vi "main.vi"() -> ()   [LabVIEW 2009]
uses:
  typedefs/ScanAxisCfg.ctl
  typedefs/AxisSelect_Enum.ctl
  typedefs/SweepMode_Ring.ctl
  typedefs/ScanType.ctl
  typedefs/DwellTime.ctl
  typedefs/PathCluster.ctl
  typedefs/main_States.ctl
  globals/VISAResourceName.vi
  typedefs/AxisSpaceCfg.ctl
  typedefs/AxisCfg.ctl
  globals/AxisSpace.vi
  typedefs/Ultra3000/Index_Numeric.ctl
  typedefs/Ultra3000/HostControlModeRing.ctl
  typedefs/Ultra3000/IndexType.ctl
  typedefs/Ultra3000/IndexSettings_Cluster.ctl
panel:
  in  "Move to index stop":bool
  in  "Move to index start":bool
  in  "Move to scan stop":bool
  in  "Move to scan start":bool
  in  "Scan Axis":T1
  in  "Same as Scan Axis":bool
  in  "Index Axis":T1={"Axis "=enum."Y", "Velocity"=0.0, "Accel./Decel."=0.0, "Deadband"=0.0, "Start Position"=0.0, "Total Length"=0.0, "Stop Position"=0.0, "Pixel Increment"=0.0}
  in  "File Paths":T3
  in  "Scan Options":T7
  in  "open":bool
  in  "Tools":T8(ring)
  in  "Exit":bool
  in  "Start Scan":bool
  # "Scan Configuration"
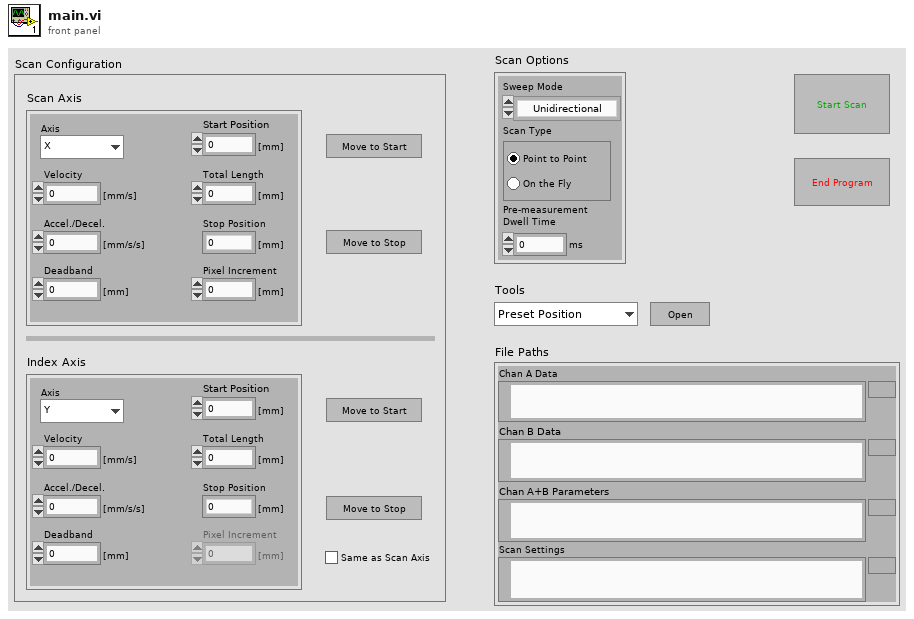
[diagram p1: front panel]
types:
  T1 = typedef "ScanAxisCfg.ctl" = cluster{"Axis ":T2, "Velocity":dbl, "Accel./Decel.":dbl, "Deadband":dbl, "Start Position":dbl, "Total Length":dbl, "Stop Position":dbl, "Pixel Increment":dbl}
  T2 = typedef "AxisSelect_Enum.ctl" = enum16{"X", "Y", "Z", "Axis Space"}
  T3 = typedef "PathCluster.ctl" = cluster{"Chan A Data":path, "Chan B Data":path, "Chan A+B Parameters":path, "Scan Settings":path}
  T4 = typedef "SweepMode_Ring.ctl" = enum16{"Unidirectional", "Bidirectional"}
  T5 = typedef "ScanType.ctl" = enum32{"Point to Point", "On the Fly"}
  T6 = typedef "DwellTime.ctl" = u16
  T7 = cluster{"Sweep Mode":T4, "Scan Type":T5, "Pre-measurement\nDwell Time":T6}
  T8 = enum16{"Preset Position", "Axis Settings", "Test Axes"}
  T9 = typedef "main_States.ctl" = enum16{"Handle FP Events", "Same as Scan Axis", "Exit", "Axis Start", "Open Tools", "Update Stop Position", "Start Scan", "Axis Stop", "Initialize Scanner", "Abort", "Connect Serial Port", "Initialize", "Export", "Import"}
  T10 = enum16{"open", "replace", "create", "open or create", "replace or create", "replace or create with confirmation"}
  T11 = typedef "Index_Numeric.ctl" = u8
  T12 = enum8{"Enabled", "Disabled", "Disabled and Grayed Out"}
  T13 = typedef "IndexSettings_Cluster.ctl" = cluster{"Type":T14, "Dwell":T6, "Velocity":dbl, "Accel/Decel":dbl}
  T14 = typedef "IndexType.ctl" = i32
  T15 = typedef "AxisSpaceCfg.ctl" = T16[]
  T16 = typedef "AxisCfg.ctl" = cluster{"Addr":u8, "Conv Factor":dbl, "Forward Limit":dbl, "Reverse Limit":dbl, "Enable Limits":bool}
  T17 = typedef "HostControlModeRing.ctl" = u16
  T18 = typedef "ReplaySettings.ctl" = cluster{"Sampling Rate":dbl, "Samples in replay":u32, "Replay Start Time":dbl, "Replay Stop Time":dbl}
  T19 = typedef "Acquire Event type.ctl" = cluster{"Acquire Mode":T20, "Acquisition mode":T21, "Acquirer":T22, "Transfer Chans":enum16{"Chan A", "Chan B", "Chan A+B"}, "A max scale":dbl, "A min scale":dbl, "B max scale":dbl, "B min scale":dbl, "A Probe":T23, "B Probe":T23, "A Coupling":T24, "B Coupling":T24, "A Bandwidth":T25, "B Bandwidth":T25, "Trigger Source":T26, "Trigger Amplitude":dbl, "A Trigger Amplitude":dbl, "B Trigger Amplitude":dbl, "Trigger Filter":T27, "Trig Slope":bool, "Trigger Holdoff":dbl, "Dig Pattern Rqd":bool, "Dig Pattern":u32, "Ext Trig Threshold":dbl, "Dig Input Threshold":dbl, "Start Time":dbl, "Stop Time":dbl, "Pre Trig Time":dbl, "Port":enum16{"Port 1", "Port 2", "Port 3", "Port 4", "Port 5", "Port 6"}, "Num divisions":i16, "Num seq frames":i16, "Num Buffers":i32, "Sig Gen Freq":dbl, "Sig Gen Amp":dbl, "Sig Gen Offset":dbl, "Sig Gen Waveform":T28, "Sig Gen Sweep":enum16{"Linear", "Log"}, "Sig Gen Func":enum16{"Standard", "Auto advance", "Freq mod In8", "Phase mod In8"}, "Sig Gen Freq 2":dbl, "Sig Gen Phase":dbl, "Trig 2 Function":T29, "Min Trigger Period":dbl, "Max trigger Period":dbl, "Trigger count":u32, "Trig 2 Slope":bool, "Trig 2 Source Chan":T30, "Trig 2 Level":dbl, "Dig Pattern 2 Rqd":bool, "Dig Pattern 2":u32, "Trigger 2 Source":enum16{"Trigger 1 inverted", "Trig 2 Defn"}, "Waveform Averages":i32, "Value changed":i32, "Freq Span":dbl, "Freq Res":dbl, "Duration":dbl, "Resolution":dbl, "Link Port":T31, "Ext Sample Clock":bool, "F Spare 2":bool, "F Spare 3":bool, "F Spare 4":bool, "Sampler Resolution":T32, "Intf Source":T33, "Update Rate":enum16{"20 Frame/sec", "10 Frame/sec", "5 Frame/sec"}, "Transfer Size":T34, "Sig Gen Freq Step":dbl, "TCP Adr":u32, "TCP port":u32, "CAU Ser Num Hi":u32, "CAU Ser Num Lo":u32, "Function Number":dbl, "Function Parameter":dbl, "Function Result":dbl, "Link Start":u32, "Link Timebase":u32, "Link Timer":u32, "Link Setup":u32, "Spare 1":dbl, "Spare 2":dbl, "Spare 3":dbl, "Spare 4":dbl}
  T20 = typedef "Acquire capture type.ctl" = enum16{"single", "automatic", "triggered", "stop", "single stop", "replay"}
  T21 = typedef "Acquire capture method.ctl" = enum16{"Sampled", "Peak Captured", "Filtered", "Repetitive", "Waveform avg"}
  T22 = typedef "Acquirer type.ctl" = enum16{"Internal Sig Gen", "APC 901", "APC 901A", "Sound Card", "Cleverscope"}
  T23 = typedef "Input Range.ctl" = enum16{"x1", "x10", "x100", "x1K", "x20", "x50", "x200"}
  T24 = typedef "Input Coupling.ctl" = enum16{"AC", "DC"}
  T25 = typedef "Input Bandwidth.ctl" = u16
  T26 = typedef "USB channel.ctl" = enum32{"Chan A", "Chan B", "Ext Trigger", "Dig Trig", "Link Input", "chan_5", "chan_6", "chan_7", "chan_8", "chan_9", "chan_10", "chan_11", "chan_12", "chan_13", "chan_14", "chan_15"}
  T27 = typedef "Trigger Filter.ctl" = enum16{"None", "Low Pass", "Hi Pass", "Noise"}
  T28 = typedef "Cscope waveform type.ctl" = enum16{"sine", "triangle", "square", "DC", "OFF"}
  T29 = typedef "Trigger Period.ctl" = enum16{"None", "Trig 1~2 < min", "min<T1~2 < max", "Trig 1~2 > max", "Count Trig 1", "Count Trig 2"}
  T30 = typedef "Trigger channel.ctl" = enum32{"Chan A", "Chan B", "Ext Trigger", "Dig Trig", "Link Input"}
  T31 = typedef "Link port types.ctl" = enum8{"Debug", "Link Out", "Disabled", "Slave", "Master", "Uart", "SPI", "I2C", "Digital", "Sig Gen"}
  T32 = typedef "Acquirer resolution.ctl" = enum16{"10 bit", "12 Bit", "14 bit"}
  T33 = typedef "Intf source.ctl" = enum16{"USB", "Ethernet - Find by IP address", "Ethernet - Find first IP address", "Ethernet - Find by serial number"}
  T34 = typedef "Acquire transfer size.ctl" = enum16{"Normal", "100% Buffer", "50% Buffer", "10% Buffer", "5% Buffer", "2% Buffer", "Sequence"}
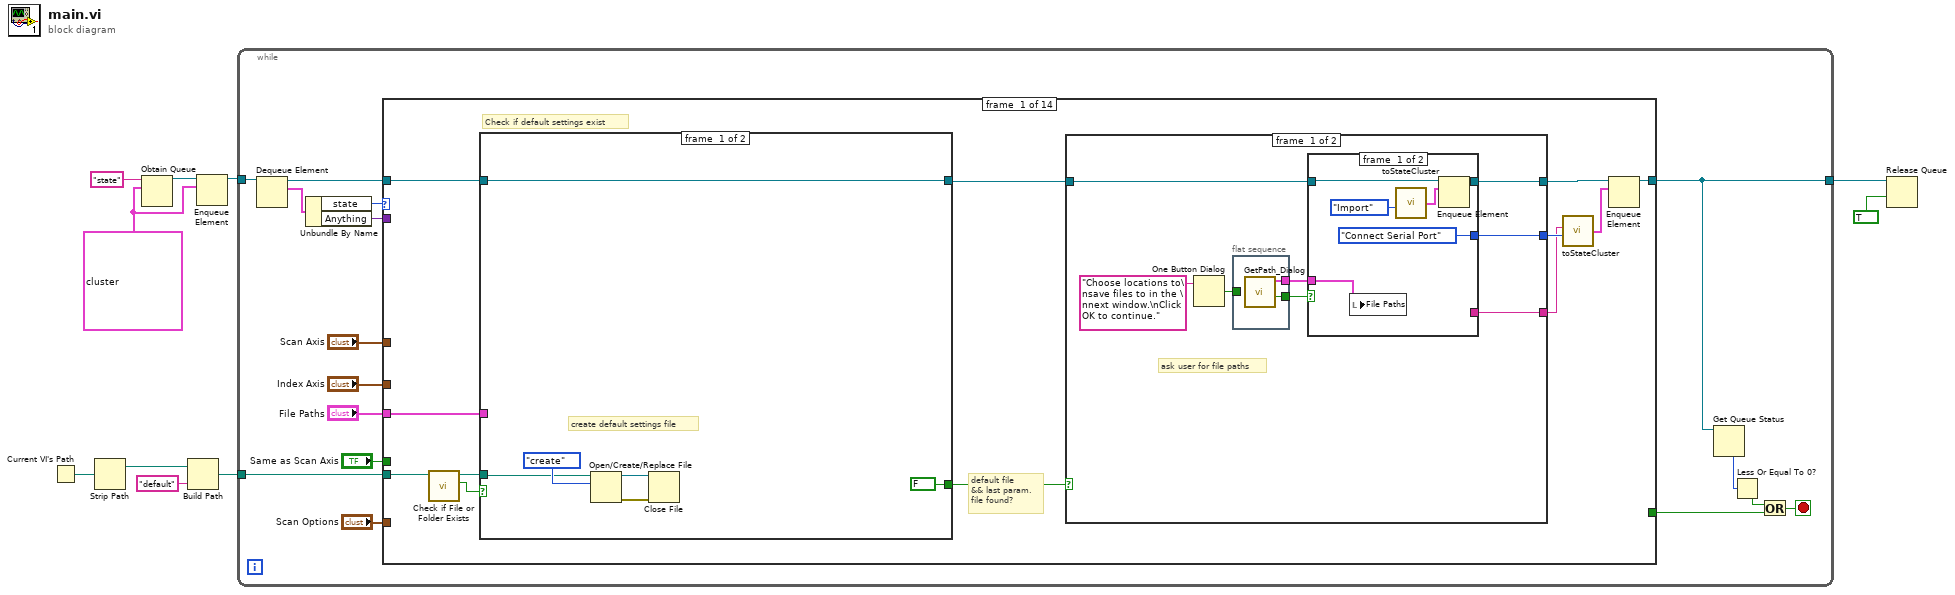
[diagram p0: block diagram]
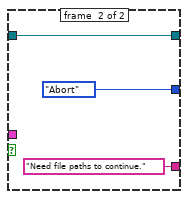
[diagram p2: hidden frame]
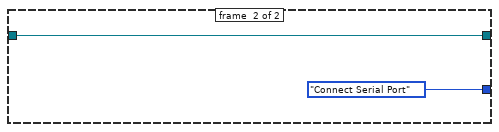
[diagram p3: hidden frame]
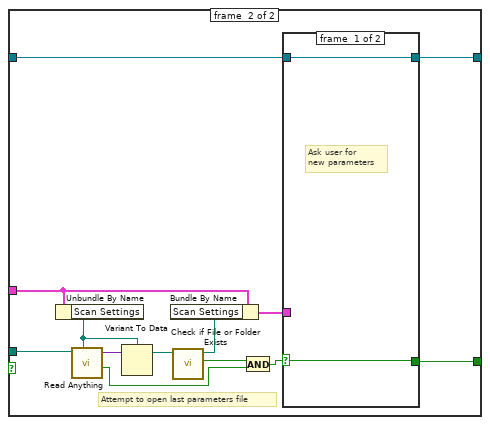
[diagram p4: hidden frame]
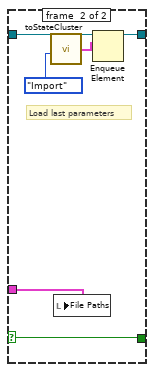
[diagram p5: hidden frame]
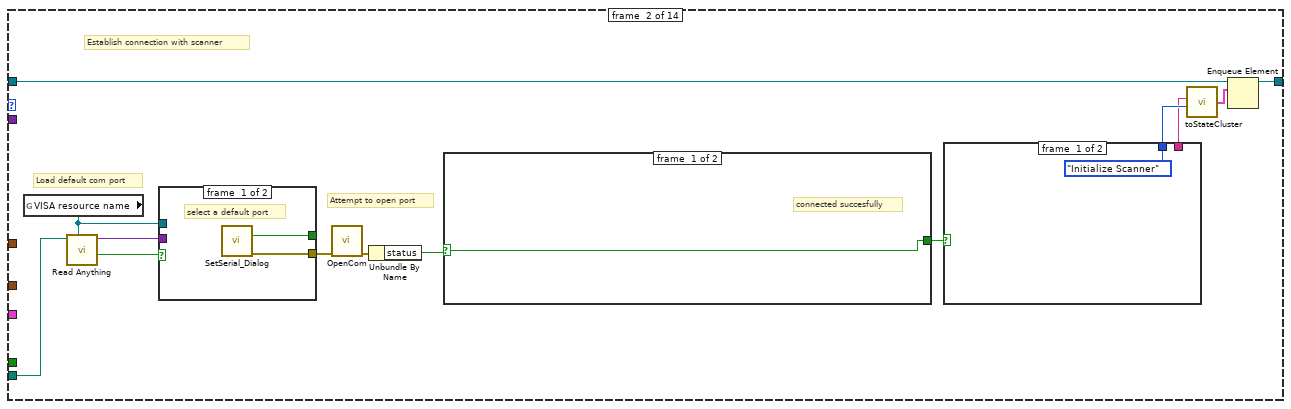
[diagram p6: hidden frame]
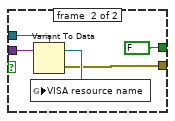
[diagram p7: hidden frame]
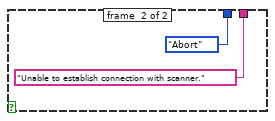
[diagram p8: hidden frame]
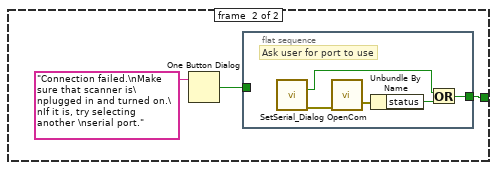
[diagram p9: hidden frame]
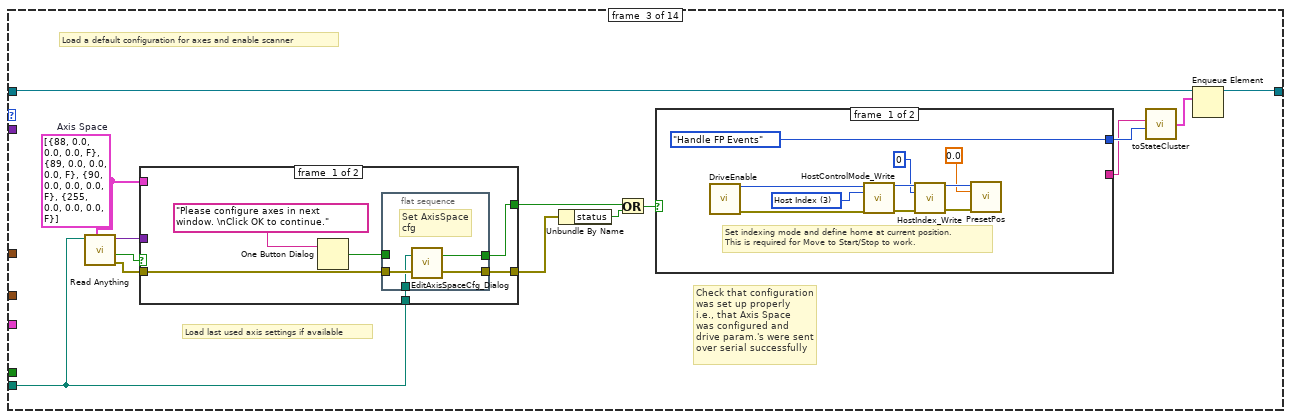
[diagram p10: hidden frame]
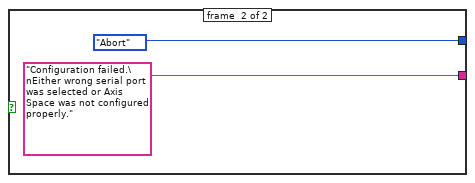
[diagram p11: hidden frame]
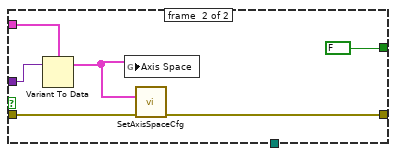
[diagram p12: hidden frame]
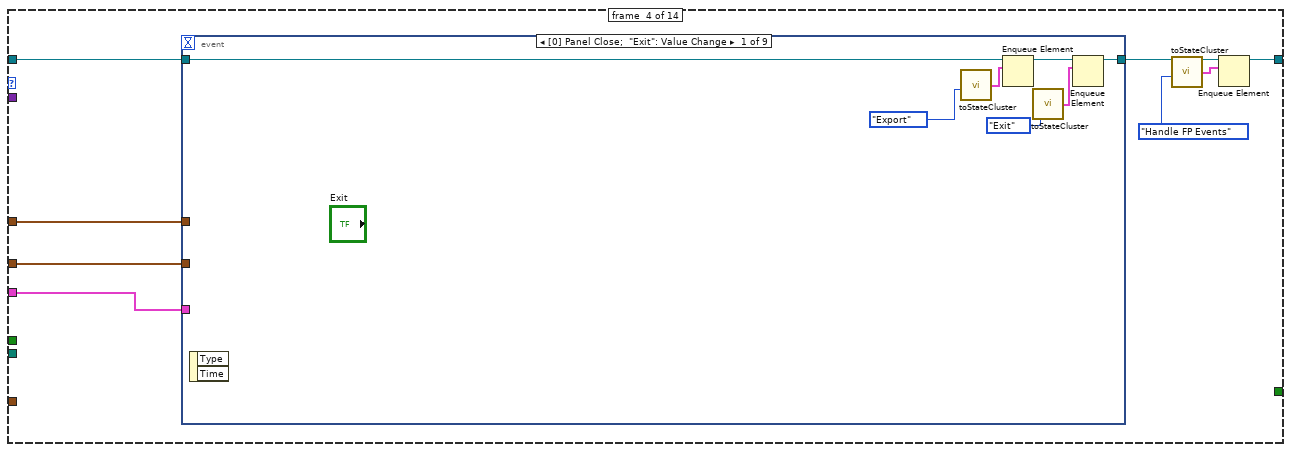
[diagram p13: hidden frame]
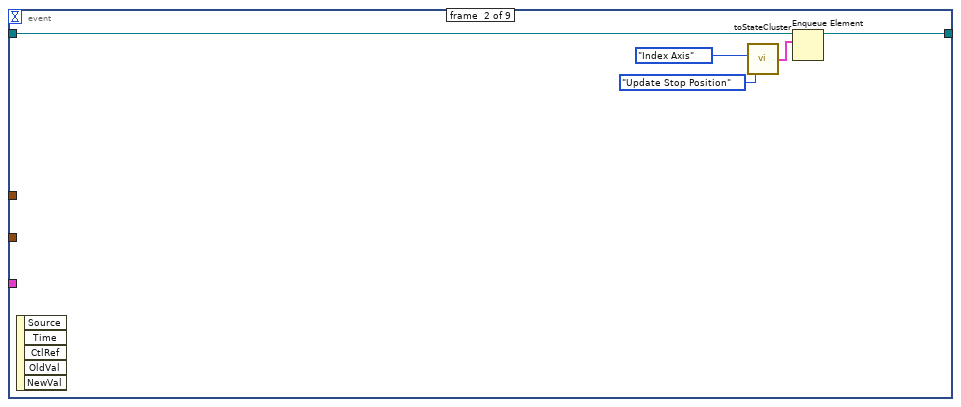
[diagram p14: hidden frame]
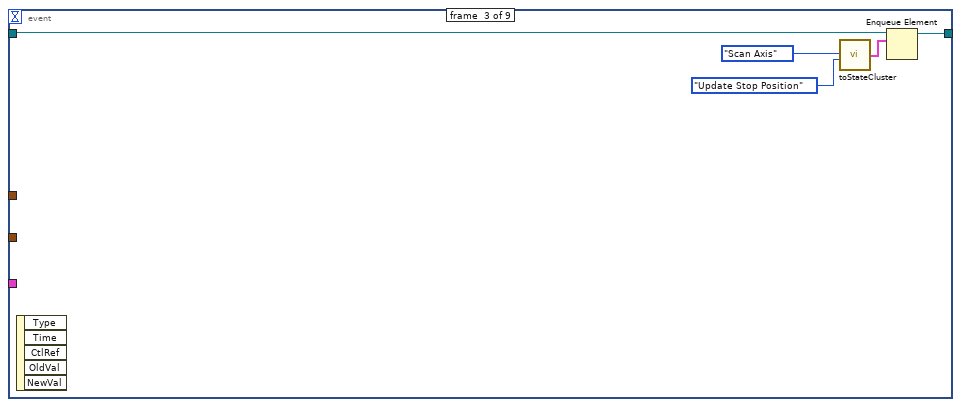
[diagram p15: hidden frame]
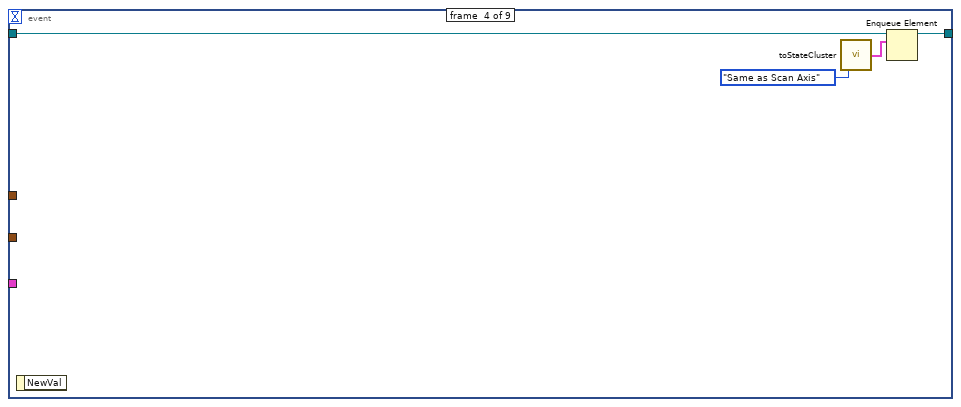
[diagram p16: hidden frame]
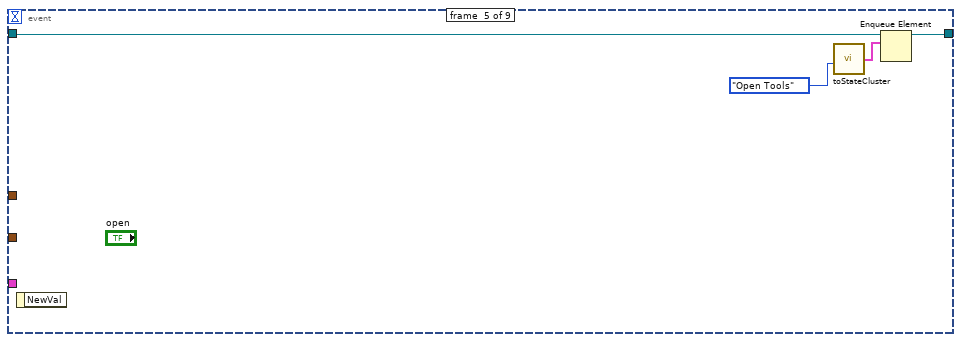
[diagram p17: hidden frame]
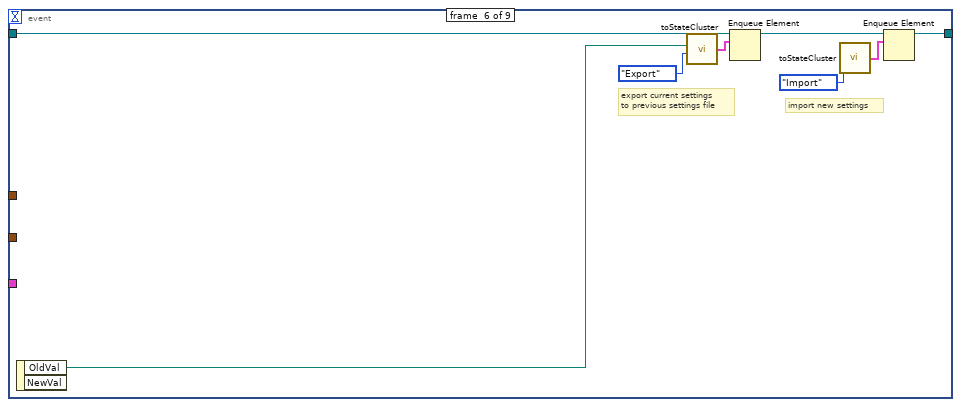
[diagram p18: hidden frame]
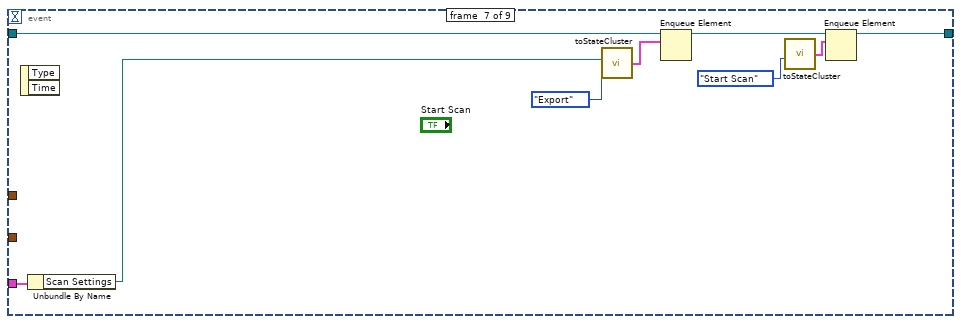
[diagram p19: hidden frame]
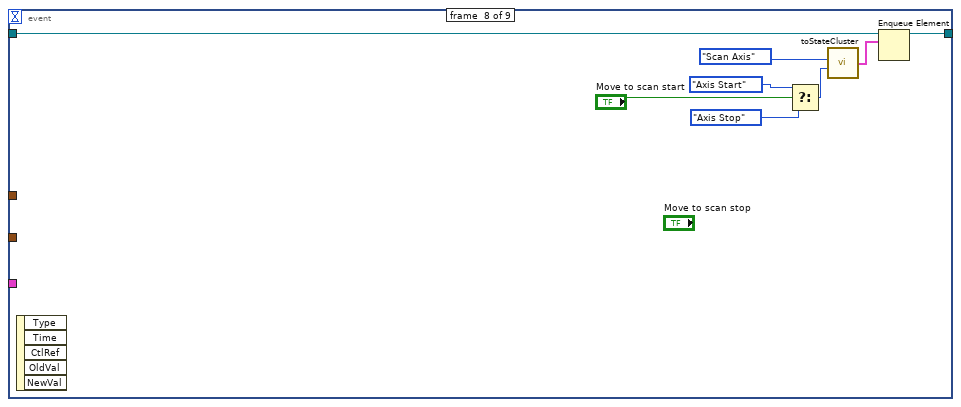
[diagram p20: hidden frame]
diagram:
  w1 = cluster{"Anything":variant, "state":T9} {"Anything"=variant, "state"=enum."Initialize"}
  n1 = Current VI's Path() -> (path=w3:path)
  n2 = Strip Path(path=w3) -> (stripped path=w2:path)  [unwired: 1 out]
  n3 = Obtain Queue(name (unnamed)="state", element data type=w1) -> (queue out=w7:refnum<queue>)  [unwired: 3 in, 2 out]
  n4 = Build Path(base path=w2, name or relative path="default") -> (appended path=w4:path)
  n5 = Enqueue Element(queue=w7, element=w1) -> (queue out=w6:refnum<queue>)  [unwired: 2 in, 2 out]
  n6 = while {
    tunnel: w6 -> [w22]
    tunnel: [w16] -> w9
    tunnel: w4 -> [w15]
    stop <- w20 stop-if-true
    n7 = Dequeue Element(queue=w22) -> (queue out=w21:refnum<queue>, element=w13:cluster{"Anything":variant, "state":T9})  [unwired: 2 in, 2 out]
    n8 = Unbundle By Name(w13) -> ("state"=w12:T9, "Anything"=w11:variant)
    n9 = case shown="\"Connect Serial Port\"" w12 {
      tunnel: "Scan Axis" -> [_ _ _ w168 w231 w244 w259 w275 _ w295 _ _ w348 w370]
      tunnel: [_ _ _ _ _ _ _ _ _ _ TRUE ("Exit") TRUE ("Exit") _ _] -> w19
      tunnel: "Index Axis" -> [_ _ _ w167 w233 _ w260 w276 _ w293 _ _ w347 w369]
      tunnel: "File Paths" -> [w36 _ _ w166 _ _ _ _ _ w294 _ w326 w340 w361]
      tunnel: "Scan Options" -> [_ _ _ _ _ _ _ _ _ w291 _ _ w346 w371]
      tunnel: w21 -> [w34 w97 w128 w165 w230 w243 w257 w273 w287 w290 w321 w329 w351 w366]
      tunnel: [w32 w98 w127 w164 w230 w243 w257 w273 w287 w290 w321 w329 w351 w367] -> w16
      tunnel: w15 -> [w38 w92 w122 _ _ _ _ _ w286 _ _ w324 _ _]
      tunnel: "Same as Scan Axis" -> [_ _ _ _ _ w242 _ _ _ _ _ _ w345 w365]
      tunnel: w11 -> [_ _ _ _ w229 _ w255 w271 _ _ w320 _ w333 w357]
      frame #0 {
        # "default file\n&& last param.\nfile found?"
        # "Check if default settings exist"
        n10 = call <vilib>:"Check if File or Folder Exists.vi"("path"=w38) -> ("file or folder exists?"=w37:bool, "dup path"=w35:path)  [unwired: 8 in, 1 out]
        n11 = case shown="True" w37 {
          tunnel: w36 -> [_ w77]
          tunnel: w35 -> [w62 w71]
          tunnel: w34 -> [w61 w72]
          tunnel: [w61 w73] -> w31
          tunnel: [FALSE w70] -> w30
          frame #0 {
            # "create default settings file"
            n12 = Open/Create/Replace File(file path (use dialog)=w62, operation (0:open)=T10."create") -> (refnum out=w64:refnum<file>, error out=w63:errorcluster)  [unwired: 4 in, 1 out]
            n13 = Close File(refnum=w64, error in=w63) -> ()  [unwired: 2 out]
          }
          frame #1 {
            # "Attempt to open last parameters file"
            n14 = Unbundle By Name(w77) -> ("Scan Settings"=w76:path)
            n15 = call "Read Anything.vi"("Type of Anything"=w76, "Path (dialog)"=w71) -> ("Found?"=w66:bool, "Anything"=w78:variant)  [unwired: 7 in, 1 out]
            n16 = Variant To Data(Variant=w78, type=w76) -> (data=w74:path)  [unwired: 1 in, 1 out]
            n17 = call <vilib>:"Check if File or Folder Exists.vi"("path"=w74) -> ("file or folder exists?"=w67:bool, "dup path"=w69:path)  [unwired: 8 in, 1 out]
            n18 = Bundle By Name(cluster=w77, "Scan Settings"=w69) -> (w75:T3)
            n19 = And(x=w67, y=w66) -> (x .and. y?=w68:bool)
            n20 = case shown="True" w68 {
              selector: w68 -> [w79 w83]
              tunnel: w75 -> [_ w86]
              tunnel: [w80 w85] -> w73
              tunnel: w72 -> [w80 w84]
              tunnel: [w79 w83] -> w70
              frame #0 {
                # "Ask user for \nnew parameters"
              }
              frame #1 {
                # "Load last parameters"
                n21 = call "toStateCluster.vi"("state"=main_States."Import" ("element")) -> ("output cluster"=w82:cluster{"Anything":variant, "state":T9})  [unwired: 5 in]
                n22 = local write "File Paths"(w86) -> ()
                n23 = Enqueue Element(queue=w84, element=w82) -> (queue out=w85:refnum<queue>)  [unwired: 2 in, 2 out]
              }
            }
          }
        }
        n24 = case shown="True" w30 {
          tunnel: [w42 _] -> w27
          tunnel: [w40 w59] -> w33
          tunnel: w31 -> [w41 w59]
          tunnel: [w39 main_States."Connect Serial Port"] -> w29
          frame #0 {
            # "ask user for file paths"
            n25 = One Button Dialog(message="Choose locations to\nsave files to in the \nnext window.\nClick OK to continue.") -> (true=w43:bool)  [unwired: 1 in]
            n26 = flat-sequence {
              tunnel: [w48] -> w46
              tunnel: [w47] -> w45
              tunnel: w43 -> [_]
              frame #0 {
                n27 = call "GetPath_Dialog.vi"() -> ("Cancelled?"=w48:bool, "File Paths Out"=w47:T3)  [unwired: 10 in]
              }
            }
            n28 = case shown="False" w46 {
              tunnel: [_ "Need file paths to continue." ("message")] -> w42
              tunnel: w45 -> [w54 _]
              tunnel: [w52 w56] -> w40
              tunnel: w41 -> [w51 w56]
              tunnel: [main_States."Connect Serial Port" main_States."Abort"] -> w39
              frame #0 {
                n29 = local write "File Paths"(w54) -> ()
                n30 = call "toStateCluster.vi"("state"=main_States."Import" ("element")) -> ("output cluster"=w50:cluster{"Anything":variant, "state":T9})  [unwired: 5 in]
                n31 = Enqueue Element(queue=w51, element=w50) -> (queue out=w52:refnum<queue>)  [unwired: 2 in, 2 out]
              }
              frame #1 {
              }
            }
          }
          frame #1 {
          }
        }
        n32 = call "toStateCluster.vi"("state"=w29, "Anything"=w27) -> ("output cluster"=w28:cluster{"Anything":variant, "state":T9})  [unwired: 4 in]
        n33 = Enqueue Element(queue=w33, element=w28) -> (queue out=w32:refnum<queue>)  [unwired: 2 in, 2 out]
      }
      frame #1 {
        # "Establish connection with scanner"
        # "Load default com port"
        # "Attempt to open port"
        n34 = global read "VISAResourceName.vi" "VISA resource name"() -> (w93:refnum<visa-resource-name>)
        n35 = call "Read Anything.vi"("Type of Anything"=w93, "Path (dialog)"=w92) -> ("Found?"=w91:bool, "Anything"=w94:variant)  [unwired: 7 in, 1 out]
        n36 = case shown="True" w91 {
          tunnel: w94 -> [_ w106]
          tunnel: w93 -> [_ w104]
          tunnel: [w101 FALSE ("Cancelled?")] -> _
          tunnel: [w100 w102] -> w90
          frame #0 {
            # "select a default port"
            n37 = call "SetSerial_Dialog.vi"() -> ("Cancelled?"=w101:bool, "error out"=w100:errorcluster)  [unwired: 14 in]
          }
          frame #1 {
            n38 = Variant To Data(Variant=w106, type=w104) -> (error out=w102:errorcluster, data=w105:refnum<visa-resource-name>)  [unwired: 1 in]
            n39 = global write "VISAResourceName.vi" "VISA resource name"(w105) -> ()
          }
        }
        n40 = call "OpenCom.vi"("error in (no error)"=w90) -> ("error out"=w96:errorcluster)  [unwired: 14 in]
        n41 = Unbundle By Name(w96) -> ("status"=w95:bool)
        n42 = case shown="True" w95 {
          selector: w95 -> [w110 _]
          tunnel: [w110 w113] -> w99
          frame #0 {
            # "connected succesfully"
          }
          frame #1 {
            n43 = One Button Dialog(message="Connection failed.\nMake sure that scanner is\nplugged in and turned on.\nIf it is, try selecting another \nserial port.") -> (true=w112:bool)  [unwired: 1 in]
            n44 = flat-sequence {
              tunnel: [w118] -> w113
              tunnel: w112 -> [_]
              frame #0 {
                # "Ask user for port to use"
                n45 = call "SetSerial_Dialog.vi"() -> ("Cancelled?"=w117:bool, "error out"=w116:errorcluster)  [unwired: 14 in]
                n46 = call "OpenCom.vi"("error in (no error)"=w116) -> ("error out"=w115:errorcluster)  [unwired: 14 in]
                n47 = Unbundle By Name(w115) -> ("status"=w114:bool)
                n48 = Or(x=w117, y=w114) -> (x .or. y?=w118:bool)
              }
            }
          }
        }
        n49 = case shown="False" w99 {
          tunnel: [main_States."Initialize Scanner" main_States."Abort"] -> w89
          tunnel: [_ "Unable to establish connection with scanner." ("message")] -> w87
          frame #0 {
          }
          frame #1 {
          }
        }
        n50 = call "toStateCluster.vi"("state"=w89, "Anything"=w87) -> ("output cluster"=w88:cluster{"Anything":variant, "state":T9})  [unwired: 4 in]
        n51 = Enqueue Element(queue=w97, element=w88) -> (queue out=w98:refnum<queue>)  [unwired: 2 in, 2 out]
      }
      frame #2 {
        w125 = T15 [{"Addr"=88, "Conv Factor"=0.0, "Forward Limit"=0.0, "Reverse Limit"=0.0, "Enable Limits"=FALSE}, {"Addr"=89, "Conv Factor"=0.0, "Forward Limit"=0.0, "Reverse Limit"=0.0, "Enable Limits"=FALSE}, {"Addr"=90, "Conv Factor"=0.0, "Forward Limit"=0.0, "Reverse Limit"=0.0, "Enable Limits"=FALSE}, {"Addr"=255, "Conv Factor"=0.0, "Forward Limit"=0.0, "Reverse Limit"=0.0, "Enable Limits"=FALSE}]  # Axis Space
        # "Load a default configuration for axes and enable scanner"
        # "Check that configuration\nwas set up properly\ni.e., that Axis Space\nwas configured and \ndrive param.'s were sent\nover serial successfully"
        # "Load last used axis settings if available"
        n52 = call "Read Anything.vi"("Type of Anything"=w125, "Path (dialog)"=w122) -> ("Error Out"=w124:errorcluster, "Found?"=w123:bool, "Anything"=w126:variant)  [unwired: 7 in]
        n53 = case shown="True" w123 {
          tunnel: [w150 FALSE ("Cancelled?")] -> w129
          tunnel: [w149 w159] -> w132
          tunnel: w124 -> [w148 w158]
          tunnel: w126 -> [_ w157]
          tunnel: w125 -> [_ w156]
          tunnel: w122 -> [w147 _]
          frame #0 {
            n54 = One Button Dialog(message="Please configure axes in next window. \nClick OK to continue.") -> (true=w145:bool)  [unwired: 1 in]
            n55 = flat-sequence {
              tunnel: [w154] -> w150
              tunnel: [w153] -> w149
              tunnel: w148 -> [w152]
              tunnel: w147 -> [w151]
              tunnel: w145 -> [_]
              frame #0 {
                # "Set AxisSpace\ncfg"
                n56 = call "EditAxisSpaceCfg_Dialog.vi"("error in"=w152, "default save path"=w151) -> ("error out"=w153:errorcluster, "Cancelled?"=w154:bool)
              }
            }
          }
          frame #1 {
            n57 = Variant To Data(Variant=w157, type=w156) -> (data=w155:T15)  [unwired: 1 in, 1 out]
            n58 = global write "AxisSpace.vi" "Axis Space"(w155) -> ()
            n59 = call "SetAxisSpaceCfg.vi"("Axis Space Config"=w155, "error in (no error)"=w158) -> ("error out"=w159:errorcluster)  [unwired: 13 in]
          }
        }
        n60 = Unbundle By Name(w132) -> ("status"=w130:bool)
        n61 = Or(x=w129, y=w130) -> (x .or. y?=w131:bool)
        n62 = case shown="False" w131 {
          tunnel: [_ "Configuration failed.\nEither wrong serial port was selected or Axis Space was not configured properly." ("message")] -> w120
          tunnel: [main_States."Handle FP Events" main_States."Abort"] -> w121
          frame #0 {
            w136 = T17 3 items=["Normal Mode", "Setpoint velocity", "Setpoint current", "Host Index"] ("Host Control Mode (Normal)")
            # "Set indexing mode and define home at current position.\nThis is required for Move to Start/Stop to work."
            n63 = call "DriveEnable.vi"() -> ("Axis Out"=w141:T2, "error out"=w135:errorcluster)  [unwired: 14 in]
            n64 = call "HostControlMode_Write.vi"("Axis In"=w141, "Host Control Mode (Normal)"=w136, "error in (no error)"=w135) -> ("Axis Out"=w137:T2, "error out"=w138:errorcluster)  [unwired: 11 in]
            n65 = call "HostIndex_Write.vi"("Axis In (Axis Space)"=w137, "Index"=T11 0, "error in (no error)"=w138) -> ("Axis Out"=w140:T2, "error out"=w139:errorcluster)  [unwired: 10 in, 1 out]
            n66 = call "PresetPos.vi"("Axis In (Axis Space)"=w140, "Preset Position"=0.0, "error in (no error)"=w139) -> ()  [unwired: 11 in, 2 out]
          }
          frame #1 {
          }
        }
        n67 = call "toStateCluster.vi"("state"=w121, "Anything"=w120) -> ("output cluster"=w119:cluster{"Anything":variant, "state":T9})  [unwired: 4 in]
        n68 = Enqueue Element(queue=w128, element=w119) -> (queue out=w127:refnum<queue>)  [unwired: 2 in, 2 out]
      }
      frame #3 {
        n69 = event shown="[0] Panel Close;  \"Exit\": Value Change" {
          selector: _ -> [_ _ _ _ _ _ _ _ _]
          dyn-events: _ -> [_ _ _ _ _ _ _ _ _]
          timeout: _ -> [_ _ _ _ _ _ _ _ _]
          tunnel: w168 -> [_ _ _ _ _ _ _ _ _]
          tunnel: w167 -> [_ _ _ _ _ _ _ _ _]
          tunnel: w166 -> [_ _ _ _ _ _ w203 _ _]
          tunnel: w165 -> [w175 w179 w184 w188 w192 w199 w208 w214 w222]
          tunnel: [w174 w180 w185 w189 w193 w201 w210 w215 w223] -> w163
          event #0 {
            n70 = event-data() -> ()  [unwired: 1 in, 2 out]
            n71 = call "toStateCluster.vi"("state"=main_States."Export") -> ("output cluster"=w172:cluster{"Anything":variant, "state":T9})  [unwired: 5 in]
            n72 = Enqueue Element(queue=w175, element=w172) -> (queue out=w173:refnum<queue>)  [unwired: 2 in, 2 out]
            n73 = call "toStateCluster.vi"("state"=main_States."Exit" ("element")) -> ("output cluster"=w170:cluster{"Anything":variant, "state":T9})  [unwired: 5 in]
            n74 = Enqueue Element(queue=w173, element=w170) -> (queue out=w174:refnum<queue>)  [unwired: 2 in, 2 out]
          }
          event #1 {
            n75 = event-data() -> ()  [unwired: 1 in, 5 out]
            n76 = call "toStateCluster.vi"("state"=main_States."Update Stop Position", "Anything"=enum16{"Scan Axis", "Index Axis"}."Index Axis") -> ("output cluster"=w178:cluster{"Anything":variant, "state":T9})  [unwired: 4 in]
            n77 = Enqueue Element(queue=w179, element=w178) -> (queue out=w180:refnum<queue>)  [unwired: 2 in, 2 out]
          }
          event #2 {
            n78 = event-data() -> ()  [unwired: 1 in, 5 out]
            n79 = call "toStateCluster.vi"("state"=main_States."Update Stop Position", "Anything"=enum16{"Scan Axis", "Index Axis"}."Scan Axis") -> ("output cluster"=w183:cluster{"Anything":variant, "state":T9})  [unwired: 4 in]
            n80 = Enqueue Element(queue=w184, element=w183) -> (queue out=w185:refnum<queue>)  [unwired: 2 in, 2 out]
          }
          event #3 {
            n81 = event-data() -> ()  [unwired: 1 in, 1 out]
            n82 = call "toStateCluster.vi"("state"=main_States."Same as Scan Axis") -> ("output cluster"=w187:cluster{"Anything":variant, "state":T9})  [unwired: 5 in]
            n83 = Enqueue Element(queue=w188, element=w187) -> (queue out=w189:refnum<queue>)  [unwired: 2 in, 2 out]
          }
          event #4 {
            n84 = event-data() -> ()  [unwired: 1 in, 1 out]
            n85 = call "toStateCluster.vi"("state"=main_States."Open Tools") -> ("output cluster"=w191:cluster{"Anything":variant, "state":T9})  [unwired: 5 in]
            n86 = Enqueue Element(queue=w192, element=w191) -> (queue out=w193:refnum<queue>)  [unwired: 2 in, 2 out]
          }
          event #5 {
            # "import new settings"
            # "export current settings\nto previous settings file"
            n87 = event-data() -> ("OldVal"=w194:path)  [unwired: 1 in, 1 out]
            n88 = call "toStateCluster.vi"("state"=main_States."Export" ("element"), "Anything"=w194) -> ("output cluster"=w196:cluster{"Anything":variant, "state":T9})  [unwired: 4 in]
            n89 = Enqueue Element(queue=w199, element=w196) -> (queue out=w200:refnum<queue>)  [unwired: 2 in, 2 out]
            n90 = call "toStateCluster.vi"("state"=main_States."Import") -> ("output cluster"=w197:cluster{"Anything":variant, "state":T9})  [unwired: 5 in]
            n91 = Enqueue Element(queue=w200, element=w197) -> (queue out=w201:refnum<queue>)  [unwired: 2 in, 2 out]
          }
          event #6 {
            n92 = event-data() -> ()  [unwired: 1 in, 2 out]
            n93 = Unbundle By Name(w203) -> ("Scan Settings"=w202:path)
            n94 = call "toStateCluster.vi"("state"=main_States."Export" ("element"), "Anything"=w202) -> ("output cluster"=w204:cluster{"Anything":variant, "state":T9})  [unwired: 4 in]
            n95 = Enqueue Element(queue=w208, element=w204) -> (queue out=w209:refnum<queue>)  [unwired: 2 in, 2 out]
            n96 = call "toStateCluster.vi"("state"=main_States."Start Scan") -> ("output cluster"=w207:cluster{"Anything":variant, "state":T9})  [unwired: 5 in]
            n97 = Enqueue Element(queue=w209, element=w207) -> (queue out=w210:refnum<queue>)  [unwired: 2 in, 2 out]
          }
          event #7 {
            n98 = event-data() -> ()  [unwired: 1 in, 5 out]
            n99 = Select(t=main_States."Axis Start", s="Move to scan start", f=main_States."Axis Stop") -> (s? t:f=w212:T9)
            n100 = call "toStateCluster.vi"("state"=w212, "Anything"=enum16{"Scan Axis", "Index Axis"}."Scan Axis") -> ("output cluster"=w213:cluster{"Anything":variant, "state":T9})  [unwired: 4 in]
            n101 = Enqueue Element(queue=w214, element=w213) -> (queue out=w215:refnum<queue>)  [unwired: 2 in, 2 out]
          }
          event #8 {
            n102 = event-data() -> ()  [unwired: 1 in, 5 out]
            n103 = Select(t=main_States."Axis Start", s="Move to index start", f=main_States."Axis Stop") -> (s? t:f=w220:T9)
            n104 = call "toStateCluster.vi"("state"=w220, "Anything"=enum16{"Scan Axis", "Index Axis"}."Index Axis") -> ("output cluster"=w219:cluster{"Anything":variant, "state":T9})  [unwired: 4 in]
            n105 = Enqueue Element(queue=w222, element=w219) -> (queue out=w223:refnum<queue>)  [unwired: 2 in, 2 out]
          }
        }
        n106 = call "toStateCluster.vi"("state"=main_States."Handle FP Events" ("element")) -> ("output cluster"=w161:cluster{"Anything":variant, "state":T9})  [unwired: 5 in]
        n107 = Enqueue Element(queue=w163, element=w161) -> (queue out=w164:refnum<queue>)  [unwired: 2 in, 2 out]
      }
      frame #4 {
        n108 = Variant To Data(Variant=w229, type=enum16{"Scan Axis", "Index Axis"}."Scan Axis") -> (data=w227:enum16{"Scan Axis", "Index Axis"})  [unwired: 1 in, 1 out]
        n109 = case shown="\"Scan Axis\", Default" w227 {
          tunnel: [w238 w239] -> w232
          tunnel: w233 -> [_ w239]
          tunnel: w231 -> [w238 _]
          frame #0 {
          }
          frame #1 {
          }
        }
        n110 = Unbundle By Name(w232) -> ("Start Position"=w237:dbl, "Total Length"=w236:dbl)
        n111 = Add(x=w237, y=w236) -> (x+y=w235:dbl)
        n112 = Bundle By Name(cluster=w232, "Stop Position"=w235) -> (w234:T1)
        n113 = case shown="\"Index Axis\"" w227 {
          tunnel: w234 -> [w240 w241]
          frame #0 {
            n114 = local write "Scan Axis"(w240) -> ()
          }
          frame #1 {
            n115 = local write "Index Axis"(w241) -> ()
          }
        }
      }
      frame #5 {
        n116 = property on="Index Axis" class="Clust (strict)"() -> ("Controls[]"=w247:refnum<vi>[])  [unwired: 2 in, 2 out]
        n117 = Unbundle By Name(w244) -> ("Pixel Increment"=w248:dbl)
        n118 = Index Array(array=w247, index=7) -> (element=w245:refnum<vi>)
        n119 = case shown="True" w242 {
          tunnel: w248 -> [w250 _]
          tunnel: w245 -> [w249 w252]
          frame #0 {
            n120 = property class="Ctl"(reference=w249, "Value"=w250, "DisabledEnum"=T12."Disabled and Grayed Out" ("Disabled")) -> ()  [unwired: 1 in, 2 out]
          }
          frame #1 {
            n121 = property class="Ctl"(reference=w252, "DisabledEnum"=T12."Enabled" ("Disabled")) -> ()  [unwired: 1 in, 2 out]
          }
        }
      }
      frame #6 {
        w261 = T14 1 items=["Incremental", "Absolute", "Registration", "Jog"] ("Type")
        n122 = Variant To Data(Variant=w255, type=enum16{"Scan Axis", "Index Axis"}."Scan Axis") -> (data=w254:enum16{"Scan Axis", "Index Axis"})  [unwired: 1 in, 1 out]
        n123 = case shown="\"Scan Axis\", Default" w254 {
          tunnel: [w268 w269] -> w258
          tunnel: w260 -> [_ w269]
          tunnel: w259 -> [w268 _]
          frame #0 {
          }
          frame #1 {
          }
        }
        n124 = Unbundle By Name(w258) -> ("Axis"=w262:T2, "Start Position"=w263:dbl, "Velocity"=w264:dbl, "Accel./Decel."=w265:dbl)
        n125 = Bundle By Name(cluster=T13 {"Type"=0, "Dwell"=0, "Velocity"=0.0, "Accel/Decel"=0.0} ("Index Settings"), "Type"=w261, "Velocity"=w264, "Accel/Decel"=w265) -> (w266:T13)
        n126 = call "SetPos.vi"("Axis In"=w262, "Position"=w263, "Index Settings"=w266) -> ()  [unwired: 10 in, 3 out]
      }
      frame #7 {
        w277 = T14 1 items=["Incremental", "Absolute", "Registration", "Jog"] ("Type")
        n127 = Variant To Data(Variant=w271, type=enum16{"Scan Axis", "Index Axis"}."Scan Axis") -> (data=w270:enum16{"Scan Axis", "Index Axis"})  [unwired: 1 in, 1 out]
        n128 = case shown="\"Scan Axis\", Default" w270 {
          tunnel: [w284 w285] -> w274
          tunnel: w276 -> [_ w285]
          tunnel: w275 -> [w284 _]
          frame #0 {
          }
          frame #1 {
          }
        }
        n129 = Unbundle By Name(w274) -> ("Axis"=w281:T2, "Stop Position"=w280:dbl, "Velocity"=w279:dbl, "Accel./Decel."=w278:dbl)
        n130 = Bundle By Name(cluster=T13 {"Type"=0, "Dwell"=0, "Velocity"=0.0, "Accel/Decel"=0.0} ("Index Settings"), "Type"=w277, "Velocity"=w279, "Accel/Decel"=w278) -> (w282:T13)
        n131 = call "SetPos.vi"("Axis In"=w281, "Position"=w280, "Index Settings"=w282) -> ()  [unwired: 10 in, 3 out]
      }
      frame #8 {
        n132 = case shown="\"Axis Settings\", Default" "Tools" {
          tunnel: w286 -> [w289 _ _]
          frame #0 {
            n133 = call "EditAxisSpaceCfg_Dialog.vi"("default save path"=w289) -> ()  [unwired: 1 in, 2 out]
          }
          frame #1 {
            n134 = call "TestAxes.vi"() -> ()  [unwired: 11 in, 1 out]
          }
          frame #2 {
            n135 = call "PresetPosition.vi"() -> ()  [unwired: 11 in, 1 out]
          }
        }
      }
      frame #9 {
        n136 = Unbundle By Name(w293) -> ("Axis"=w296:T2)
        n137 = Unbundle By Name(w295) -> ("Axis"=w297:T2)
        n138 = Not Equal?(x=w297, y=w296) -> (x != y?=w292:bool)
        n139 = case shown="True" w292 {
          tunnel: w293 -> [_ w307]
          tunnel: w295 -> [_ w308]
          tunnel: w294 -> [_ w300]
          tunnel: w291 -> [_ w299]
          frame #0 {
            n140 = One Button Dialog(message="Scan and Index axis must be unique") -> ()  [unwired: 1 in, 1 out]
          }
          frame #1 {
            n141 = Unbundle By Name(w300) -> ("Scan Settings"=w301:path)
            n142 = call "Acquisition_Dialog.vi"("Scan Parameters file path"=w301) -> ("Replay settings out"=w305:T18, "Acquisition Unit Out"=w303:i32, "Acquire Defn Out"=w304:T19, "Cancelled?"=w302:bool, "error out"=w306:errorcluster)  [unwired: 10 in]
            n143 = case shown="False" w302 {
              tunnel: w308 -> [w314 _]
              tunnel: w307 -> [w313 _]
              tunnel: w306 -> [w310 _]
              tunnel: w305 -> [w315 _]
              tunnel: w304 -> [w316 _]
              tunnel: w303 -> [w317 _]
              tunnel: w300 -> [w312 _]
              tunnel: w299 -> [w311 _]
              frame #0 {
                # "ignore error"
                n144 = call "Scan_Dialog.vi"("Acquisition Unit in (0)"=w317, "Acquire Definition"=w316, "Replay settings"=w315, "File Paths"=w312, "Scan Options"=w311, "error in"=w310, "Scan Axis Config"=w314, "Index Axis Config"=w313) -> ("error out"=w309:errorcluster)  [unwired: 7 in]
                n145 = Unbundle By Name(w309) -> ()  [unwired: 1 out]
              }
              frame #1 {
              }
            }
          }
        }
      }
      frame #10 {
        # "Abort message"
        n146 = Variant To Data(Variant=w320, type="" ("message")) -> (data=w318:string)  [unwired: 1 in, 1 out]
        n147 = One Button Dialog(message=w318) -> (true=w323:bool)  [unwired: 1 in]
        n148 = flat-sequence {
          tunnel: w323 -> [_]
          frame #0 {
            n149 = Stop() -> ()  [unwired: 1 in]
          }
        }
      }
      frame #11 {
        # "Write default settings file"
        # "Close serial communications with the scanner"
        # "Disable axes"
        n150 = Unbundle By Name(w326) -> ("Scan Settings"=w325:path)
        n151 = global read "VISAResourceName.vi" "VISA resource name"() -> (w328:refnum<visa-resource-name>)
        n152 = call "Write Anything.vi"("Anything"=w325, "Path (dialog)"=w324) -> ("Error Out"=w327:errorcluster)  [unwired: 9 in]
        n153 = call "Write Anything.vi"("Error In"=w327, "Anything"=w328, "Path (dialog)"=w324) -> ()  [unwired: 8 in, 1 out]
        n154 = call "DriveEnable.vi"("Enable (T)"=FALSE) -> ("error out"=w332:errorcluster)  [unwired: 13 in, 1 out]
        n155 = call "CloseCom.vi"("error in (no error)"=w332) -> ()  [unwired: 14 in, 1 out]
      }
      frame #12 {
        # "export to scan settings path by default"
        n156 = call "isVariantEmpty.vi"("Anything"=w333) -> ("empty?"=w334:bool)  [unwired: 4 in]
        n157 = case shown="True" w334 {
          tunnel: [w353 path "" ("stripped path")] -> w337
          tunnel: w333 -> [w352 _]
          frame #0 {
            n158 = Variant To Data(Variant=w352, type=path "" ("stripped path")) -> (data=w353:path)  [unwired: 1 in, 1 out]
          }
          frame #1 {
          }
        }
        n159 = Unbundle By Name(w340) -> ("Scan Settings"=w336:path)
        n160 = Empty String/Path?(string/path=w337) -> (empty?=w339:bool)
        n161 = Not(x=w339) -> (.not. x?=w338:bool)
        n162 = Select(t=w337, s=w338, f=w336) -> (s? t:f=w335:path)
        n163 = call "Write Anything.vi"("Anything"=w340, "Path (dialog)"=w335) -> ("Error Out"=w350:errorcluster)  [unwired: 9 in]
        n164 = property on="Index Axis" class="Clust (strict)"() -> ("Label.Text"=w342:string)  [unwired: 2 in, 2 out]
        n165 = call "Write Anything.vi"("Error In"=w350, "Anything"=w346, "Path (dialog)"=w335) -> ("Error Out"=w343:errorcluster)  [unwired: 8 in]
        n166 = property on="Scan Axis" class="Clust (strict)"() -> ("Label.Text"=w341:string)  [unwired: 2 in, 2 out]
        n167 = call "Write Anything.vi"("Error In"=w343, "Section Name (Name of \"Anything\")"=w342, "Anything"=w347, "Path (dialog)"=w335) -> ("Error Out"=w349:errorcluster)  [unwired: 7 in]
        n168 = call "Write Anything.vi"("Error In"=w349, "Section Name (Name of \"Anything\")"=w341, "Anything"=w348, "Path (dialog)"=w335) -> ("Error Out"=w344:errorcluster)  [unwired: 7 in]
        n169 = call "Write Anything.vi"("Error In"=w344, "Anything"=w345, "Path (dialog)"=w335) -> ()  [unwired: 8 in, 1 out]
      }
      frame #13 {
        # "import from scan settings path by default"
        n170 = call "isVariantEmpty.vi"("Anything"=w357) -> ("empty?"=w358:bool)  [unwired: 4 in]
        n171 = Unbundle By Name(w361) -> ("Scan Settings"=w360:path)
        n172 = case shown="True" w358 {
          tunnel: [w373 path "" ("stripped path")] -> w356
          tunnel: w357 -> [w372 _]
          frame #0 {
            n173 = Variant To Data(Variant=w372, type=path "" ("stripped path")) -> (data=w373:path)  [unwired: 1 in, 1 out]
          }
          frame #1 {
          }
        }
        n174 = Empty String/Path?(string/path=w356) -> (empty?=w363:bool)
        n175 = Not(x=w363) -> (.not. x?=w362:bool)
        n176 = Select(t=w356, s=w362, f=w360) -> (s? t:f=w359:path)
        n177 = Empty String/Path?(string/path=w359) -> (empty?=w364:bool)
        n178 = case shown="False" w364 {
          tunnel: w371 -> [w395 _]
          tunnel: w370 -> [w391 _]
          tunnel: w369 -> [w388 _]
          tunnel: w361 -> [w384 _]
          tunnel: w359 -> [w382 _]
          tunnel: [w380 FALSE ("Same as Scan Axis")] -> w368
          tunnel: w365 -> [w379 _]
          frame #0 {
            n179 = call "Read Anything.vi"("Type of Anything"=w384, "Path (dialog)"=w382) -> ("Error Out"=w397:errorcluster, "Anything"=w386:variant)  [unwired: 7 in, 1 out]
            n180 = Variant To Data(Variant=w386, type=w384) -> (data=w385:T3)  [unwired: 1 in, 1 out]
            n181 = local write "File Paths"(w385) -> ()
            n182 = property on="Index Axis" class="Clust (strict)"() -> ("Label.Text"=w376:string)  [unwired: 2 in, 2 out]
            n183 = call "Read Anything.vi"("Type of Anything"=w388, "Error In"=w397, "Section Name (Name of \"Type of Anything\")"=w376, "Path (dialog)"=w382) -> ("Error Out"=w396:errorcluster, "Anything"=w389:variant)  [unwired: 5 in, 1 out]
            n184 = Variant To Data(Variant=w389, type=w388) -> (data=w387:T1)  [unwired: 1 in, 1 out]
            n185 = local write "Index Axis"(w387) -> ()
            n186 = property on="Scan Axis" class="Clust (strict)"() -> ("Label.Text"=w378:string)  [unwired: 2 in, 2 out]
            n187 = call "Read Anything.vi"("Type of Anything"=w391, "Error In"=w396, "Section Name (Name of \"Type of Anything\")"=w378, "Path (dialog)"=w382) -> ("Error Out"=w377:errorcluster, "Anything"=w392:variant)  [unwired: 5 in, 1 out]
            n188 = Variant To Data(Variant=w392, type=w391) -> (data=w390:T1)  [unwired: 1 in, 1 out]
            n189 = local write "Scan Axis"(w390) -> ()
            n190 = call "Read Anything.vi"("Type of Anything"=w395, "Error In"=w377, "Path (dialog)"=w382) -> ("Error Out"=w381:errorcluster, "Anything"=w394:variant)  [unwired: 6 in, 1 out]
            n191 = Variant To Data(Variant=w394, type=w395) -> (data=w393:T7)  [unwired: 1 in, 1 out]
            n192 = local write "Scan Options"(w393) -> ()
            n193 = call "Read Anything.vi"("Type of Anything"=w379, "Error In"=w381, "Path (dialog)"=w382) -> ("Anything"=w383:variant)  [unwired: 6 in, 2 out]
            n194 = Variant To Data(Variant=w383, type=w379) -> (data=w380:bool)  [unwired: 1 in, 1 out]
            n195 = local write "Same as Scan Axis"(w380) -> ()
          }
          frame #1 {
          }
        }
        n196 = case shown="True" w368 {
          tunnel: [w399 w403] -> w367
          tunnel: w366 -> [w399 w402]
          frame #0 {
          }
          frame #1 {
            n197 = call "toStateCluster.vi"("state"=main_States."Same as Scan Axis" ("element")) -> ("output cluster"=w401:cluster{"Anything":variant, "state":T9})  [unwired: 5 in]
            n198 = Enqueue Element At Opposite End(queue=w402, element=w401) -> (queue out=w403:refnum<queue>)  [unwired: 2 in, 2 out]
          }
        }
      }
    }
    n199 = Get Queue Status(queue=w16) -> (# elements in queue=w17:i32)  [unwired: 2 in, 7 out]
    n200 = Less Or Equal To 0?(x=w17) -> (x <= 0?=w18:bool)
    n201 = Or(x=w18, y=w19) -> (x .or. y?=w20:bool)
  }
  n202 = Release Queue(queue=w9, force destroy? (F)=TRUE) -> ()  [unwired: 1 in, 3 out]
